vi "Read.vi"(8 "error in (no error)":errorcluster, 9 "timeout ms (25000)":i32, 10 "# bytes to read":i32, 11 "OpenSSL Socket in":refnum<class "SSL Socket.lvclass">) -> (0 "error out":errorcluster, 2 "Read Bytes":u8[](array[numeric]), 3 "OpenSSL Socket out":refnum<class "SSL Socket.lvclass">)   [LabVIEW 2013, in "OpenSSL Socket.lvlib" / "SSL Socket.lvclass"]
doc: "Reads data from a socket connection.\nWebSockets 2.0.0.28\nSam Sharp - MediaMongrels Ltd\nCopyright (c) 2019, MediaMongrels Ltd"
uses:
  SSL Socket.lvclass
  SSL Socket.lvclass/SSL Socket.ctl
  SSL_Lib/BIO/BIO.lvclass
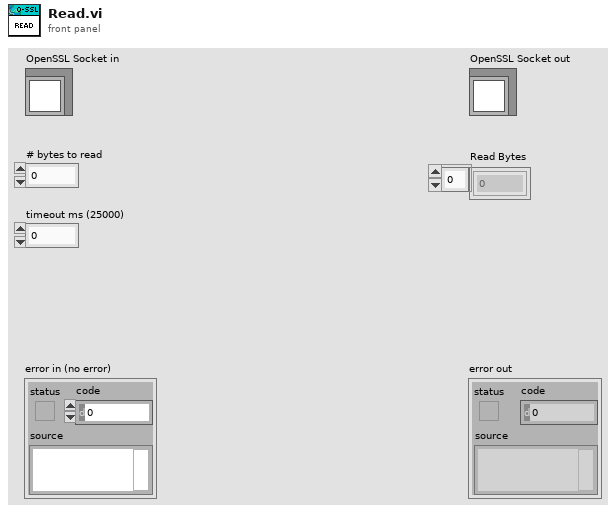
[diagram p1: front panel]
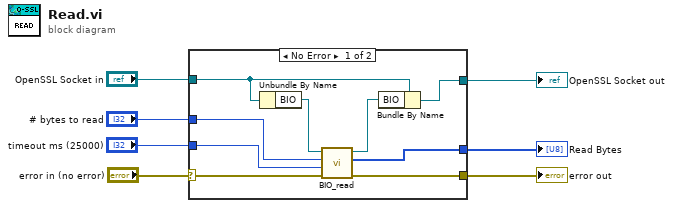
[diagram p0: block diagram]
diagram:
  n1 = case shown="No Error" "error in (no error)" {
    selector: "error in (no error)" -> [w10 w17]
    tunnel: [w16 w17] -> w4
    tunnel: "# bytes to read" -> [w8 _]
    tunnel: "timeout ms (25000)" -> [w9 _]
    tunnel: "OpenSSL Socket in" -> [w14 w18]
    tunnel: [w12 w18] -> w6
    tunnel: [w11 _] -> w3
    frame No Error {
      n2 = Unbundle By Name(w14) -> ("BIO"=w15:refnum<class "BIO.lvclass">)
      n3 = call "BIO_read.vi"("error in (no error)"=w10, "Timeout (10000ms)"=w9, "bytes to read"=w8, "BIO in"=w15) -> ("error out"=w16:errorcluster, "Bytes read"=w11:u8[], "BIO out"=w13:refnum<class "BIO.lvclass">)  [unwired: 5 in]
      n4 = Bundle By Name(cluster=w14, "BIO"=w13) -> (w12:refnum<class "SSL Socket.lvclass">)
    }
    frame Error {
    }
  }
  "error out" <- w4
  "OpenSSL Socket out" <- w6
  "Read Bytes" <- w3
